vi "BAP2F.vi"() -> ()   [LabVIEW 2014]
doc: "exp sim BAP2F\n\nDisplays acquisition graph and an analysis graph which can be fine-tuned by the user. This then can export the fitting parameters into a .txt file and saved in an appropriate directory. \n\nSubvis Used:\nDamp Sine Fit BAP2b, Damp Sine Wave Gen\n\nBeverly Abadines\nPHY 350\nBAP2F"
uses:
  typedefs/measurment parameters.ctl
  typedefs/damped wave parameter cluster.ctl
  <vilib>/Utility/file.llb/Write To Spreadsheet File (DBL).vi
panel:
  in  "Stop":bool
  in  "Save Data":bool
  out "Data to Save":dbl[][](array[numeric])
  in  "Fitting Parameters":T1={"amplitude (V)"=8.0, "frequency (Hz)"=10000.0, "start phase (deg)"=45.0, "decay rate (1/sec)"=10000.0} {"decay rate (1/sec)" scale=0.0..20000.0; "start phase (deg)" scale=-180.0..180.0; "frequency (Hz)" scale=0.0..20000.0; "amplitude (V)" scale=0.0..10.0}
  out "Analysis Graph":cluster{dbl[], "time array out (s)":dbl[]}[](graph)
  out "Acquisition Graph":T2(graph)
  out "count":i32
  in  "Measurement Parameters":T3={"time step (s)"=1e-06, "N meas"=500, "N meas reps"=100}
  in  "Start":bool
  # "Simulated Experiment"
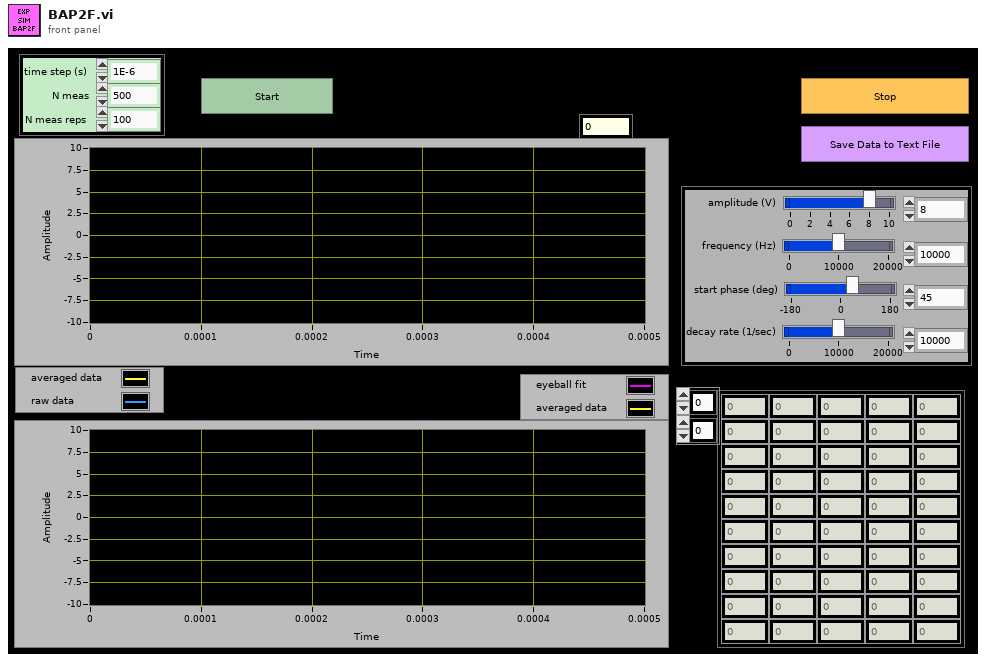
[diagram p1: front panel]
types:
  T1 = typedef "damped wave parameter cluster.ctl" = cluster{"amplitude (V)":dbl, "frequency (Hz)":dbl, "start phase (deg)":dbl, "decay rate (1/sec)":dbl}
  T2 = cluster{"time array (s)":dbl[], "voltage array (V)":dbl[]}[]
  T3 = typedef "measurment parameters.ctl" = cluster{"time step (s)":dbl, "N meas":i32, "N meas reps":i32}
  T4 = cluster{"time array (s)":dbl[], "voltage array (V)":dbl[]}
  T5 = cluster{"time array out (s)":dbl[], "voltage array out (V)":dbl[]}
  T6 = cluster{"time array out (s)":dbl[], "voltage array out (V)":dbl[]}[]
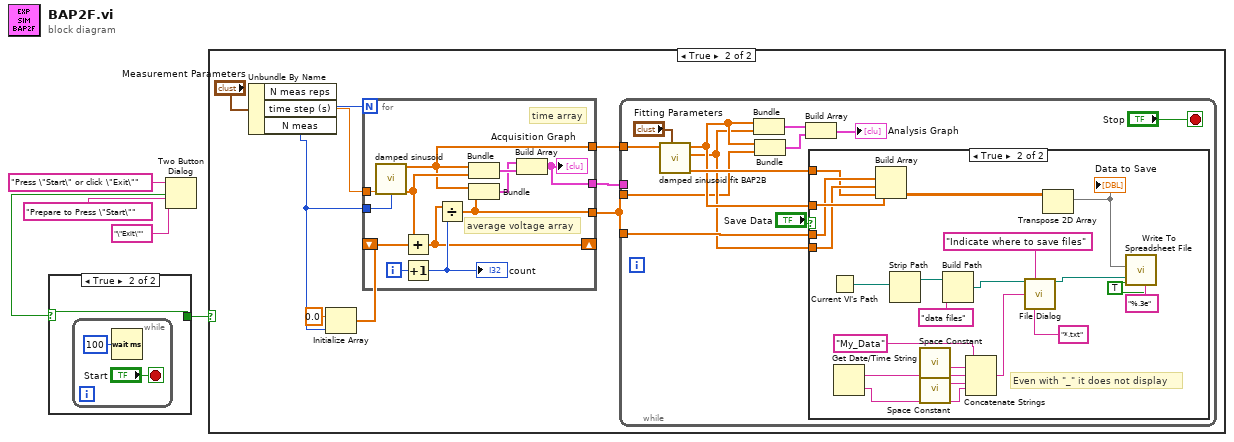
[diagram p0: block diagram]
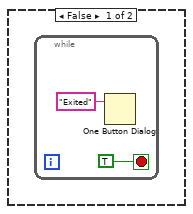
[diagram p3: hidden frame]
diagram:
  n1 = Two Button Dialog(message="Press \"Start\" or click \"Exit\"", 1:"\"Exit\"" ("F button name (\"Cancel\")"), 2:"Prepare to Press \"Start\"" ("T button name (\"OK\")")) -> (T button?=w2:bool)
  n2 = case shown="True" w2 {
    selector: w2 -> [w6 w7]
    tunnel: [w6 w7] -> w1
    frame False {
    }
    frame True {
      n3 = while {
        stop <- "Start" stop-if-true
        n4 = Wait (ms)(milliseconds to wait=u32 100) -> ()  [unwired: 1 out]
      }
    }
  }
  n5 = case shown="True" w1 {
    frame False {
      n6 = while {
        stop <- TRUE stop-if-true
        n7 = One Button Dialog(message="Exited") -> ()  [unwired: 1 in, 1 out]
      }
    }
    frame True {
      n8 = Unbundle By Name("Measurement Parameters") -> ("N meas reps"=w15:i32, "time step (s)"=w19:dbl, "N meas"=w16:i32)
      n9 = Initialize Array(0.0 ("element"), w16) -> (w18:dbl[])
      n10 = for {
        N: w15 -> [_]
        tunnel: w19 -> [w65]
        tunnel: w16 -> [w64]
        shift-right: [w59] -> _
        shift-left: w18 -> [w60]
        tunnel: [w56] -> w14
        tunnel: [w55] -> w12
        tunnel: [w54] -> w13
        i -> [w63]
        # "average voltage array"
        # "time array"
        n11 = call "damped sinusoid.vi"("time step (s)"=w65, "N meas"=w64) -> ("time array (s)"=w56:dbl[], "voltage array (V)"=w61:dbl[])  [unwired: 12 in]
        n12 = Add(x=w61, y=w60) -> (x+y=w59:dbl[])
        n13 = Increment(x=w63) -> (x+1=w62:i32)
        "count" <- w62
        n14 = Divide(x=w59, y=w62) -> (x/y=w55:dbl[])
        n15 = Bundle("time array (s)"=w56, "voltage array (V)"=w61) -> (w58:T4)  [unwired: 1 in]
        n16 = Bundle("time array (s)"=w56, w55) -> (w57:cluster{"time array (s)":dbl[], dbl[]})  [unwired: 1 in]
        n17 = Build Array(w57, w58) -> (w54:T2)
        "Acquisition Graph" <- w54
      }
      n18 = while {
        tunnel: w14 -> [w32]
        tunnel: w12 -> [w21]
        tunnel: w13 -> [_]
        tunnel: w12 -> [w26]
        stop <- "Stop" stop-if-true
        n19 = call "damped sinusoid fit BAP2B.vi"("fitting parameters"="Fitting Parameters", "time array in (s)"=w32) -> ("parameters array out"=w25:dbl[], "voltage array out (V)"=w22:dbl[], "time array out (s)"=w23:dbl[])  [unwired: 7 in]
        n20 = Bundle("time array out (s)"=w23, "voltage array out (V)"=w22) -> (w29:T5)  [unwired: 1 in]
        n21 = Bundle("time array out (s)"=w23, w21) -> (w24:cluster{"time array out (s)":dbl[], dbl[]})  [unwired: 1 in]
        n22 = Build Array(w29, w24) -> (→"Analysis Graph":T6)
        n23 = case shown="True" "Save Data" {
          tunnel: w23 -> [_ w52]
          tunnel: w26 -> [_ w51]
          tunnel: w22 -> [_ w50]
          tunnel: w25 -> [_ w49]
          frame False {
            # "Do Nothing"
          }
          frame True {
            w46 = TRUE
            # "Even with \"_\" it does not display"
            n24 = Current VI's Path() -> (path=w39:path)
            n25 = Get Date/Time String() -> (date string=w43:string, time string=w45:string)  [unwired: 1 in, 2 out]
            n26 = Build Array(w52, w51, w50, w49) -> (w53:dbl[][])
            n27 = Strip Path(path=w39) -> (stripped path=w41:path)  [unwired: 1 out]
            n28 = call <vilib>:"Space Constant.vi"() -> ("String"=w42:string)
            n29 = call <vilib>:"Space Constant.vi"() -> ("String"=w44:string)
            n30 = Build Path(base path=w41, name or relative path="data files") -> (appended path=w38:path)
            n31 = Concatenate Strings("My_Data", w42, w43, w44, w45) -> (w33:string)
            n32 = call "File Dialog"("start path"=w38, "prompt"="Indicate where to save files" ("prompt (Choose or enter file path)"), "default name"=w33, "pattern (all files)"="*.txt" ("pattern")) -> ("selected path"=w36:path)  [unwired: 8 in, 3 out]
            n33 = Transpose 2D Array(2D array=w53) -> (transposed array=w47:dbl[][])
            "Data to Save" <- w47
            n34 = call-poly <vilib>:"Write To Spreadsheet File.vi"("transpose? (no:F)"=w46, "format (%.3f)"="%.3e", "append to file? (new file:F)"=w46, "2D data"=w47, "file path (dialog if empty)"=w36) -> ()  [unwired: 3 in, 1 out]
          }
        }
      }
    }
  }
